vi "Main.vi"(8 "error in":errorcluster, 11 "MainUI in":refnum<class "MainUI.lvclass">) -> (0 "error out":errorcluster, 3 "MainUI out":refnum<class "MainUI.lvclass">)   [LabVIEW 2019, in "MainUI.lvclass"]
doc: "The <b>Queued Message Handler</b> of the Worker that owns this VI."
uses:
  MainUI.lvclass
  MainUI.lvclass/MainUI.ctl
  Initialization Data.ctl
  Response Cases.ctl
  rql_CallMAGetMeasureData.ctl
  rql_CallMBGetMeterValue.ctl
  rql_CallMCGetDIOStatus.ctl
  ModuleA/ModuleA.lvclass
  ModuleB/ModuleB.lvclass
  ModuleC/ModuleC.lvclass
  rql_UpdatePanel.ctl
  rql_SchduleABC.ctl
  rql_SchduleCAB.ctl
  rql_SchduleBCA.ctl
panel:
  in  "B>C>A":bool
  in  "C>A>B":bool
  in  "A>B>C":bool
  in  "ReadDIO":bool
  in  "ReadMeter":bool
  in  "ReadWaveform":bool
  out "DIOStatus":bool[](array[boolean])
  out "Meter":dbl(knob) scale=20.0..30.0
  out "Waveform Graph":waveform(dbl)(graph)
  # "讓各module 自我讀取最新數值 \n在MainUI 呼叫要求時回報最後的數據"
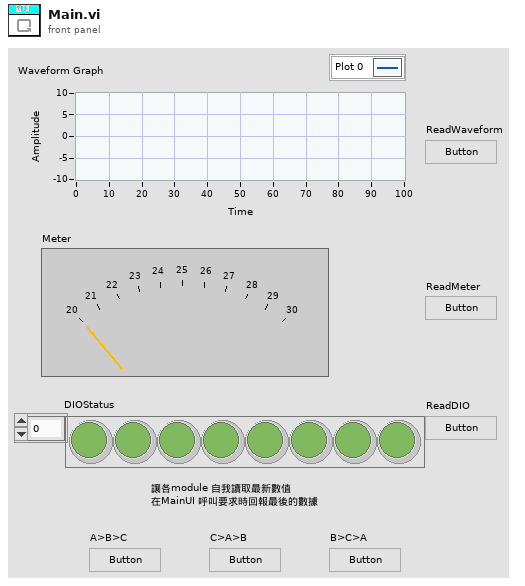
[diagram p1: front panel]
types:
  T1 = typedef "MainUI.lvclass/Initialization Data.ctl" = cluster{"Response Cases":T2}
  T2 = typedef "MainUI.lvclass/Response Cases.ctl" = cluster{"Placeholder - Can be deleted":string}
  T3 = typedef "MainUI.lvclass/rql_CallMAGetMeasureData.ctl" = cluster{"String":string}
  T4 = typedef "MainUI.lvclass/rql_CallMBGetMeterValue.ctl" = cluster{"String":string}
  T5 = typedef "MainUI.lvclass/rql_CallMCGetDIOStatus.ctl" = cluster{"String":string}
  T6 = typedef "MainUI.lvclass/rql_UpdatePanel.ctl" = cluster{"String":string}
  T7 = typedef "MainUI.lvclass/rql_SchduleABC.ctl" = cluster{"String":string}
  T8 = typedef "MainUI.lvclass/rql_SchduleCAB.ctl" = cluster{"String":string}
  T9 = typedef "MainUI.lvclass/rql_SchduleBCA.ctl" = cluster{"String":string}
  T10 = typedef "ModuleA.lvclass/rwr_RequestMeasureData Reply.ctl" = cluster{"String":string, "Waveform":waveform(dbl)}
  T11 = typedef "ModuleB.lvclass/rwr_RequestMeterValue Reply.ctl" = cluster{"String":string, "MeterValue":dbl}
  T12 = typedef "ModuleC.lvclass/rwr_RequestDIOStatus Reply.ctl" = cluster{"String":string, "DIOStatus":bool[]}
  T13 = typedef "ModuleA.lvclass/rsp_FeedbackMA_Data.ctl" = cluster{"String":string, "Waveform":waveform(dbl)}
  T14 = typedef "ModuleB.lvclass/rsp_ReturnMeterValue.ctl" = cluster{"String":string, "MeterValue":dbl}
  T15 = typedef "ModuleC.lvclass/rsp_ReturnDIOStatus.ctl" = cluster{"String":string, "DIOStatus":bool[]}
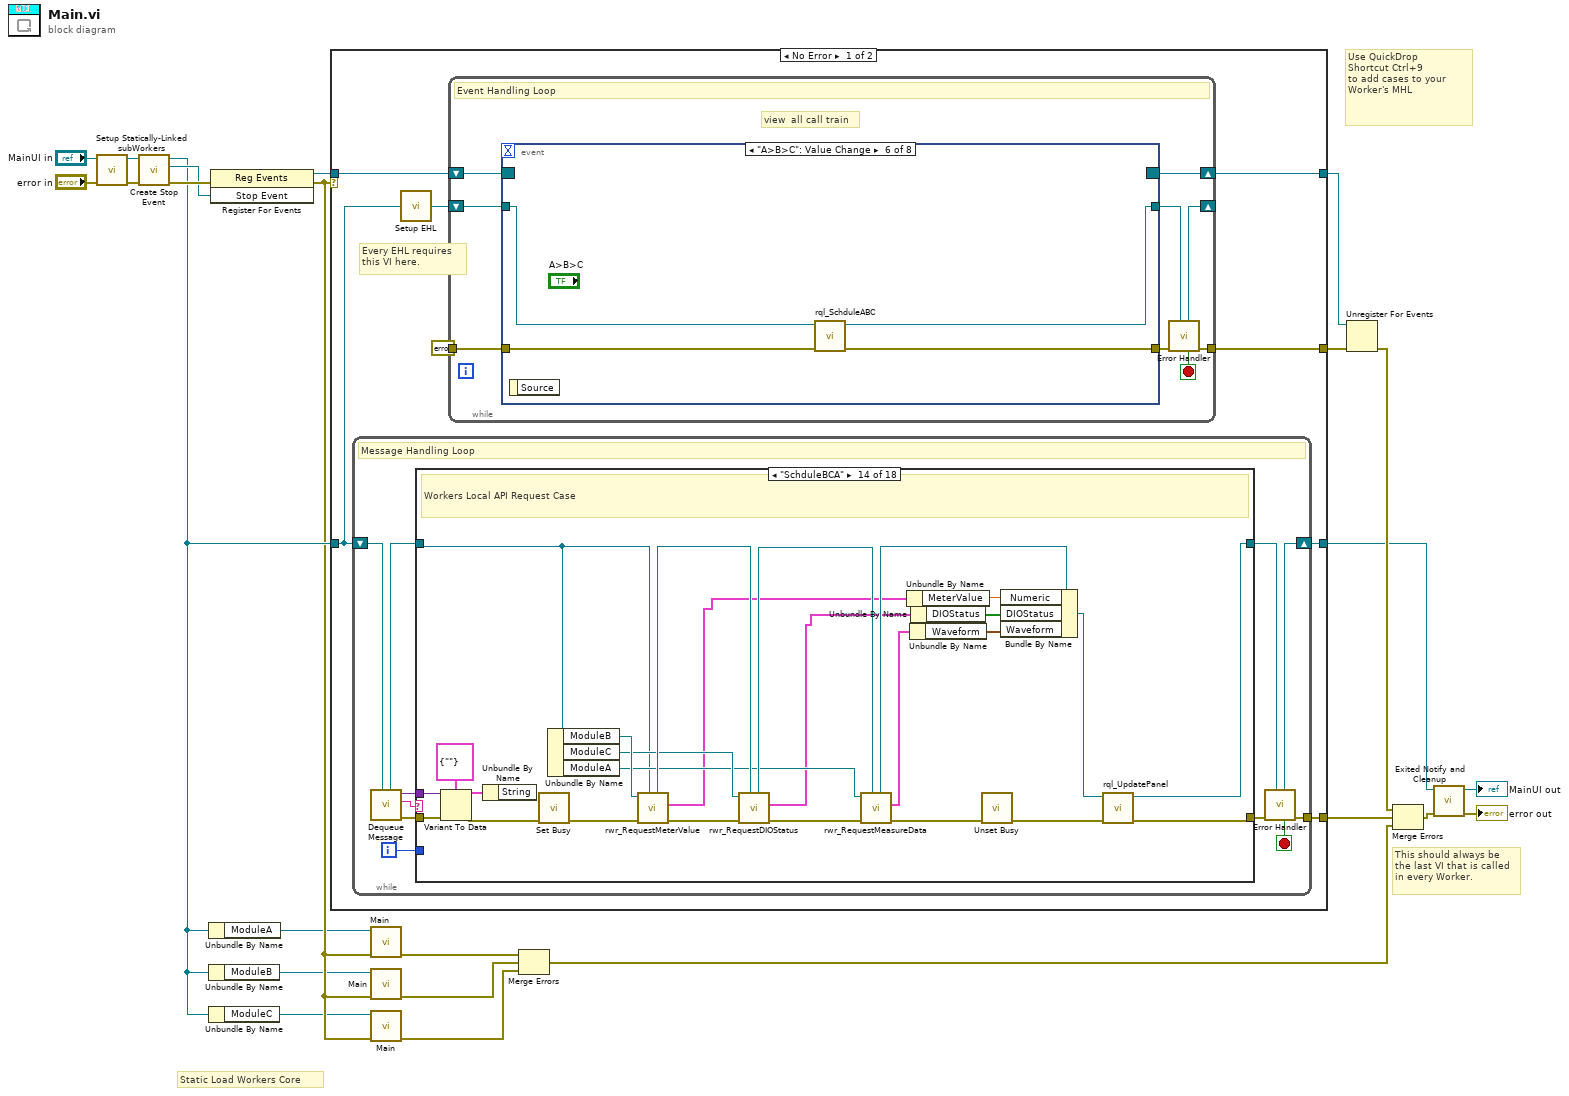
[diagram p0: block diagram]
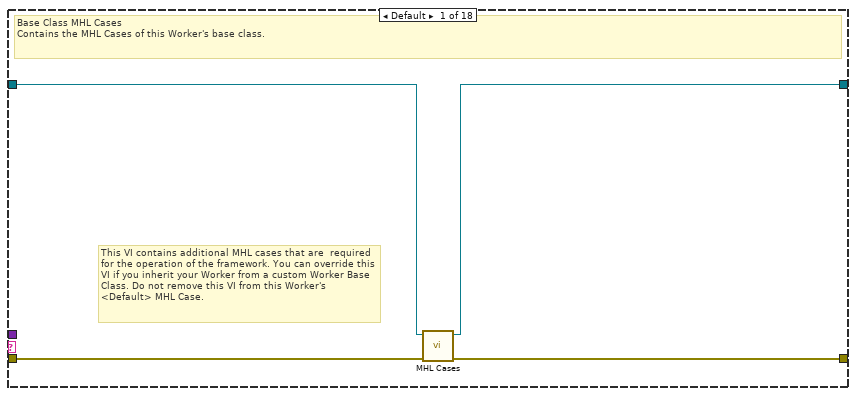
[diagram p2: hidden frame]
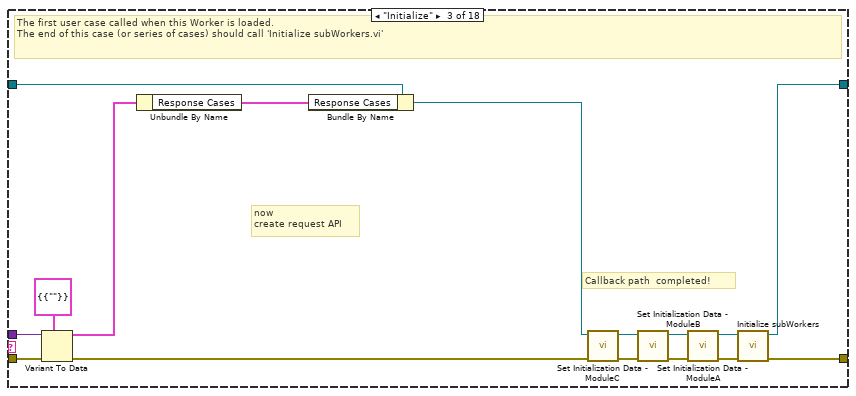
[diagram p4: hidden frame]
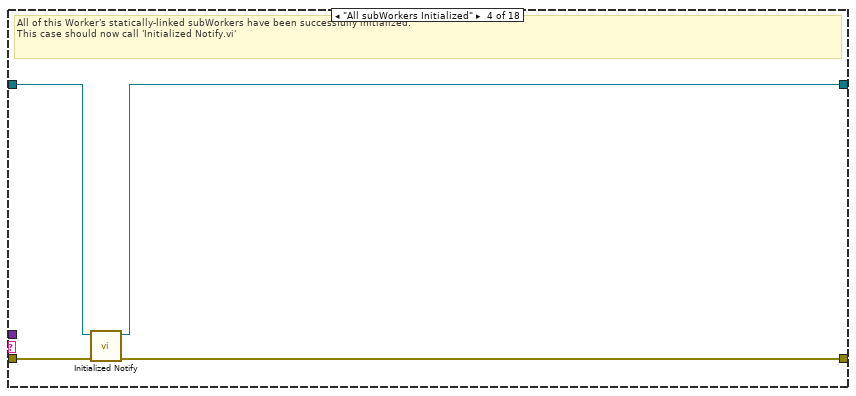
[diagram p5: hidden frame]
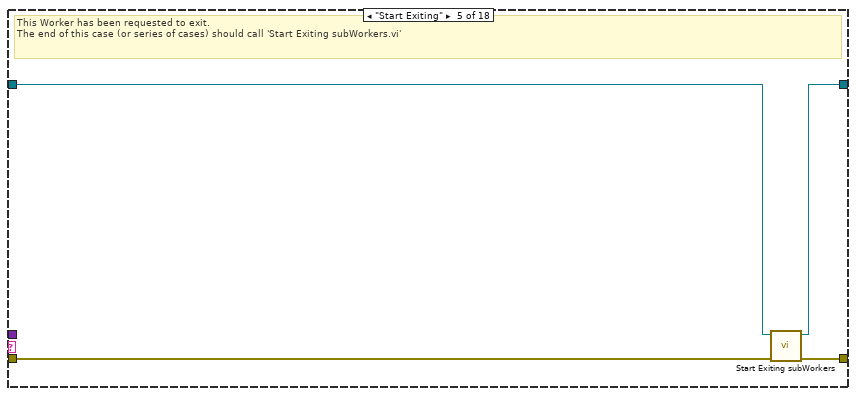
[diagram p6: hidden frame]
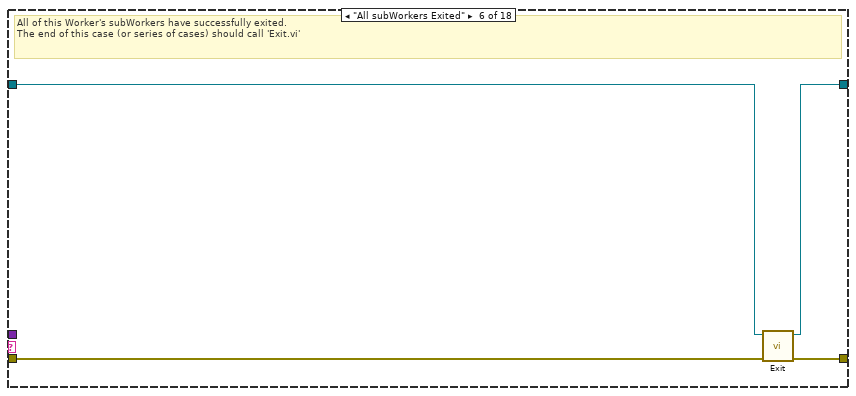
[diagram p7: hidden frame]
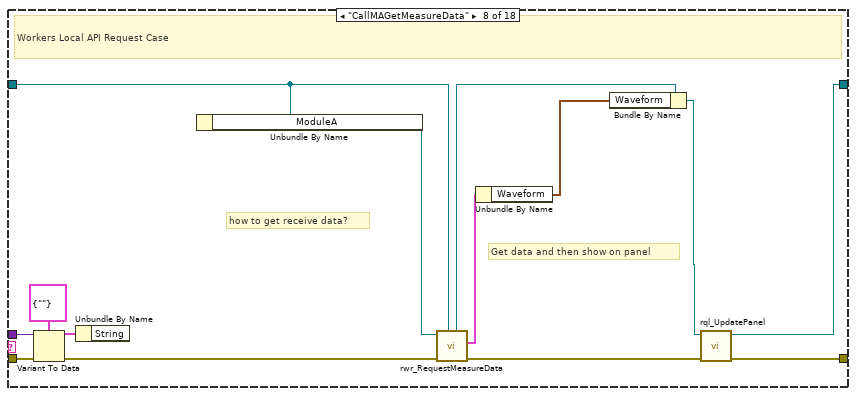
[diagram p9: hidden frame]
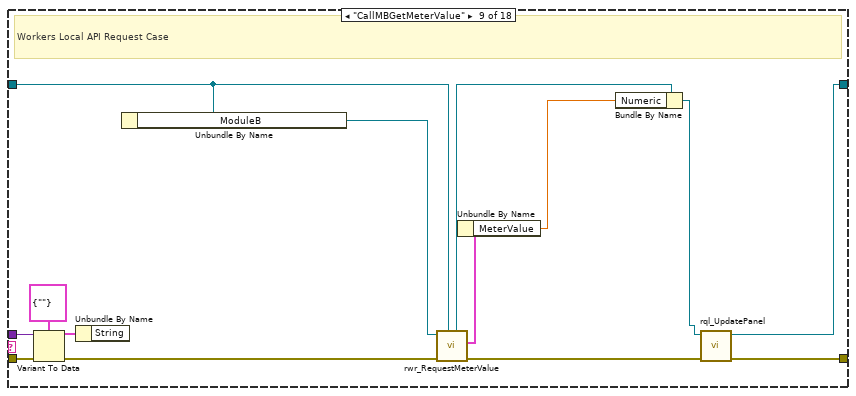
[diagram p10: hidden frame]
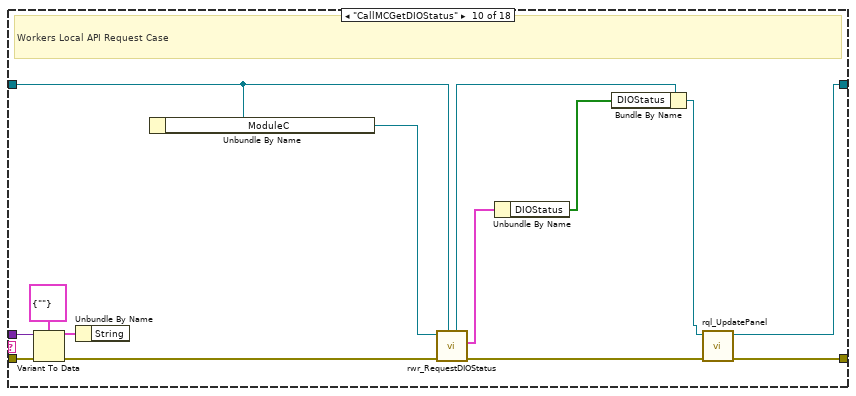
[diagram p11: hidden frame]
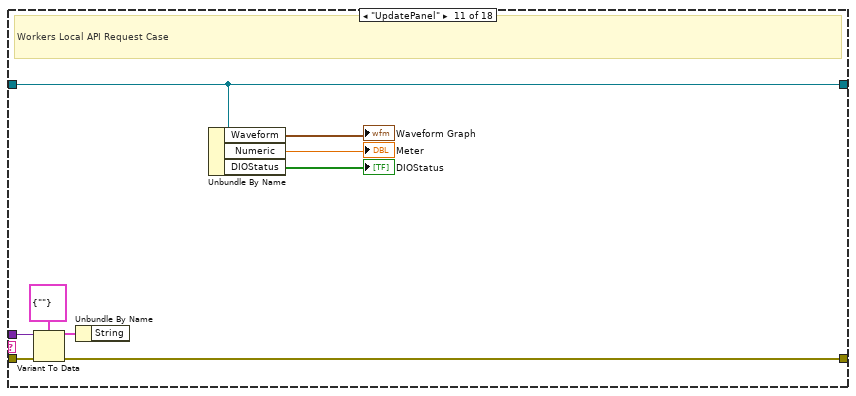
[diagram p12: hidden frame]
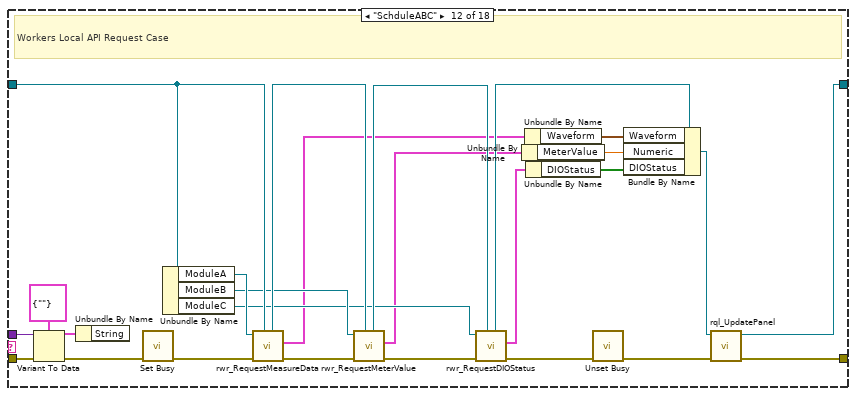
[diagram p13: hidden frame]
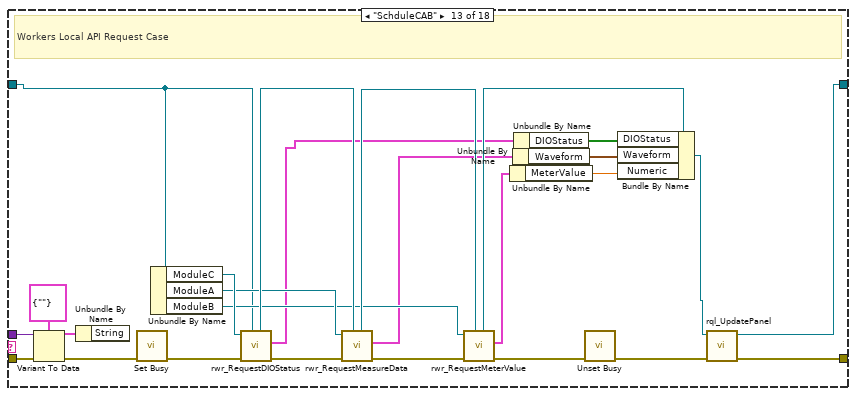
[diagram p14: hidden frame]
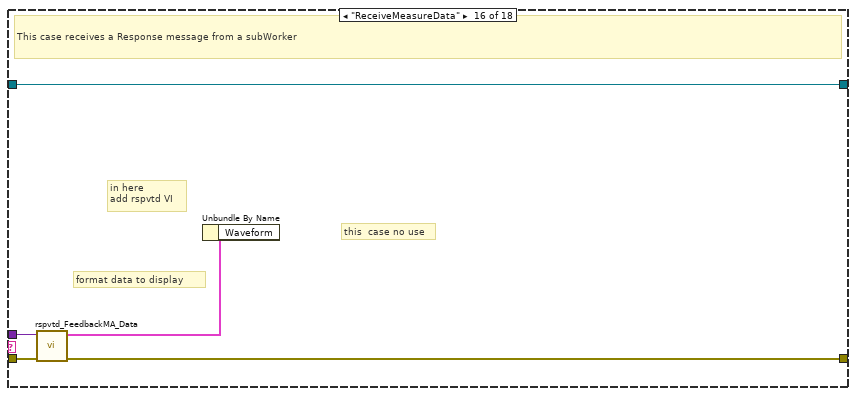
[diagram p16: hidden frame]
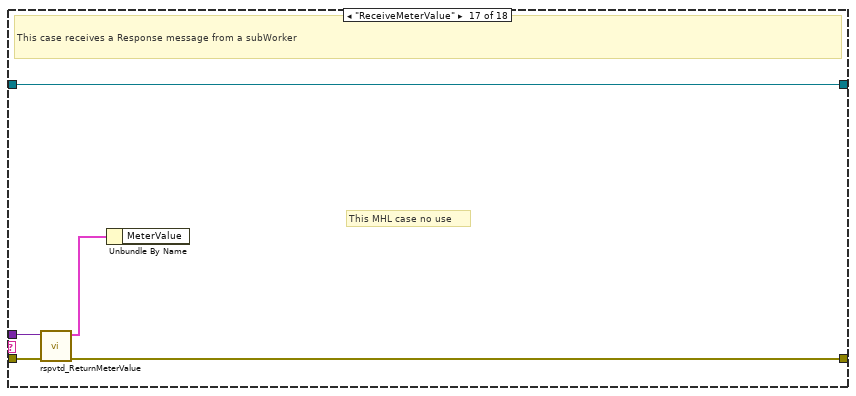
[diagram p17: hidden frame]
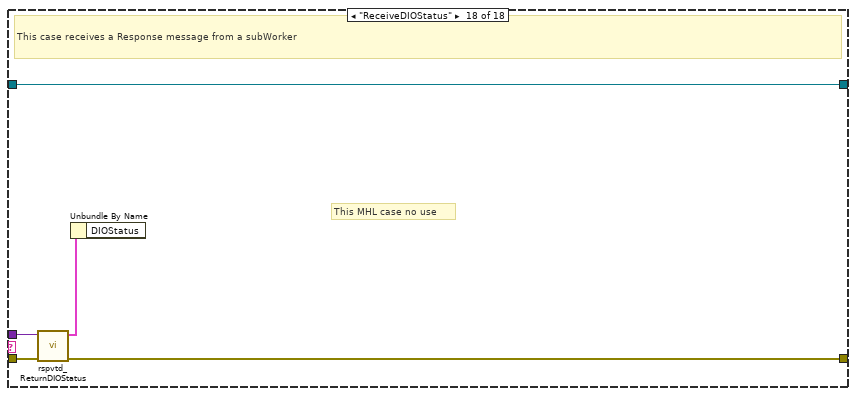
[diagram p18: hidden frame]
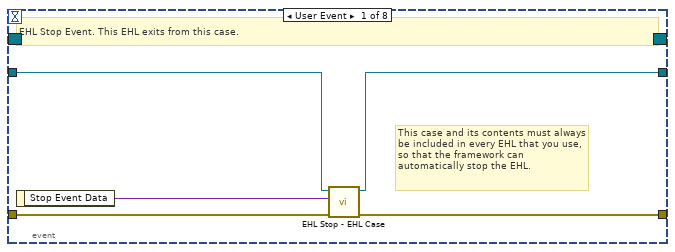
[diagram p19: hidden frame]
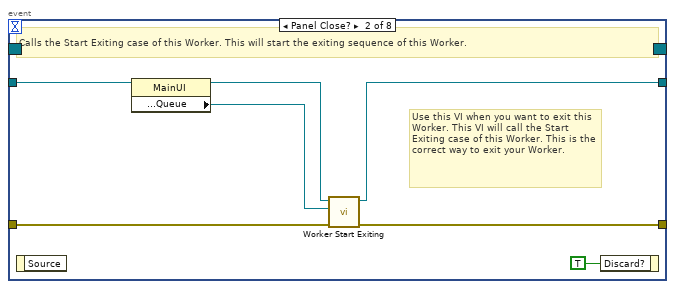
[diagram p20: hidden frame]
diagram:
  # "Static Load Workers Core"
  # "Use QuickDrop\nShortcut Ctrl+9\nto add cases to your\nWorker's MHL"
  # "This should always be the last VI that is called in every Worker."
  n1 = call "Setup Statically-Linked subWorkers.vi"("error in"="error in", "MainUI in"="MainUI in") -> ("error out"=w10:errorcluster, "MainUI out"=w8:refnum<class "MainUI.lvclass">)  [unwired: 8 in]
  n2 = call-dynamic "Create Stop Event.vi"("error in"=w10, "Worker"=w8) -> ("error out"=w19:errorcluster, "Stop Event"=w16:refnum<user-event>, "Worker out"=w13:refnum<class "MainUI.lvclass">)  [unwired: 7 in]
  n3 = Unbundle By Name(w13) -> ("ModuleA"=w5:refnum<class "ModuleA.lvclass">)
  n4 = Unbundle By Name(w13) -> ("ModuleB"=w3:refnum<class "ModuleB.lvclass">)
  n5 = Unbundle By Name(w13) -> ("ModuleC"=w1:refnum<class "ModuleC.lvclass">)
  n6 = register-events(error in=w19, w16) -> (reference out=w18:refnum<event-registration>, error out=w11:errorcluster)  [unwired: 1 in]
  n7 = case shown="No Error" w11 {
    tunnel: w13 -> [w27 w272]
    tunnel: [w25 w273] -> w17
    tunnel: w18 -> [w32 w274]
    tunnel: [w29 w275] -> w23
    tunnel: [w31 w274] -> w22
    tunnel: [w26 w271] -> w20
    selector: w11 -> [_ w275]
    frame No Error {
      # "Every EHL requires\nthis VI here."
      n8 = while {
        shift-right: [w41] -> w26
        shift-left: w27 -> [w43]
        tunnel: [w42] -> w25
        i -> [w34]
        stop <- w35 stop-if-true
        # "Message Handling Loop"
        n9 = call-dynamic "Dequeue Message.vi"("Worker"=w43) -> ("error out"=w40:errorcluster, "Case out"=w36:string, "Data out"=w33:variant, "Worker out"=w38:refnum<class "MainUI.lvclass">)  [unwired: 6 in, 1 out]
        n10 = case "Worker MHL Case Structure (DO NOT CHANGE LABEL NAME)" shown="\"SchduleBCA\"" w36 {
          tunnel: w40 -> [w47 w48 w63 w67 w70 w77 w79 w93 w107 w121 w130 w156 w182 w208 w210 w215 w220 w225]
          tunnel: [w46 w48 w65 w66 w73 w76 w79 w82 w96 w110 w129 w135 w161 w187 w210 w213 w218 w223] -> w39
          tunnel: w38 -> [w45 w49 w62 w69 w71 w75 w78 w86 w100 w114 w125 w150 w170 w196 w209 w214 w219 w224]
          tunnel: [w44 w49 w64 w68 w72 w74 w78 w80 w94 w108 w125 w133 w159 w185 w209 w214 w219 w224] -> w37
          tunnel: w34 -> [_ _ _ _ _ _ _ _ _ _ _ _ _ _ _ _ _ _]
          tunnel: w33 -> [_ _ w60 _ _ _ _ w90 w104 w118 w127 w153 w180 w206 _ w212 w217 w222]
          frame Default {
            # "This VI contains additional MHL cases that are  required for the operation of the framework. You can override this VI if you inherit your Worker from a custom Worker Base Class. Do not remove this VI from this Worker's <Default> MHL Case."
            # "Base Class MHL Cases\nContains the MHL Cases of this Worker's base class."
            n11 = call-dynamic "MHL Cases.vi"("error in"=w47, "Worker in"=w45) -> ("error out"=w46:errorcluster, "Worker out"=w44:refnum<class "MainUI.lvclass">)  [unwired: 8 in]
          }
          frame "------------ FRAMEWORK CASES -----------" {
            # "Start of Workers Framework Cases"
          }
          frame "Initialize" {
            # "now \ncreate request API"
            # "Callback path  completed!"
            # "The first user case called when this Worker is loaded.\nThe end of this case (or series of cases) should call 'Initialize subWorkers.vi'"
            n12 = Variant To Data(error in=w63, type=T1 {"Response Cases"={"Placeholder - Can be deleted"=""}} ("Initialization Data"), Variant=w60) -> (data=w59:T1, error out=w61:errorcluster)
            n13 = Unbundle By Name(w59) -> ("Response Cases"=w58:T2)
            n14 = Bundle By Name(cluster=w62, "Response Cases"=w58) -> (w51:refnum<class "MainUI.lvclass">)
            n15 = call "Set Initialization Data - ModuleC.vi"("error in"=w61, "MainUI in"=w51) -> ("error out"=w52:errorcluster, "MainUI out"=w50:refnum<class "MainUI.lvclass">)  [unwired: 8 in]
            n16 = call "Set Initialization Data - ModuleB.vi"("error in"=w52, "MainUI in"=w50) -> ("error out"=w54:errorcluster, "MainUI out"=w53:refnum<class "MainUI.lvclass">)  [unwired: 8 in]
            n17 = call "Set Initialization Data - ModuleA.vi"("error in"=w54, "MainUI in"=w53) -> ("error out"=w56:errorcluster, "MainUI out"=w55:refnum<class "MainUI.lvclass">)  [unwired: 8 in]
            n18 = call-dynamic "Initialize subWorkers.vi"("error in"=w56, "Worker"=w55) -> ("error out"=w65:errorcluster, "dup Worker out"=w64:refnum<class "MainUI.lvclass">)  [unwired: 8 in]
          }
          frame "All subWorkers Initialized" {
            # "All of this Worker's statically-linked subWorkers have been successfully initialized.\nThis case should now call 'Initialized Notify.vi'"
            n19 = call-dynamic "Initialized Notify.vi"("error in"=w67, "Worker"=w69) -> ("error out"=w66:errorcluster, "dup Worker out"=w68:refnum<class "MainUI.lvclass">)  [unwired: 8 in]
          }
          frame "Start Exiting" {
            # "This Worker has been requested to exit. \nThe end of this case (or series of cases) should call 'Start Exiting subWorkers.vi'"
            n20 = call-dynamic "Start Exiting subWorkers.vi"("error_in"=w70, "Worker"=w71) -> ("error out"=w73:errorcluster, "dup Worker out"=w72:refnum<class "MainUI.lvclass">)  [unwired: 8 in]
          }
          frame "All subWorkers Exited" {
            # "All of this Worker's subWorkers have successfully exited. \nThe end of this case (or series of cases) should call 'Exit.vi'"
            n21 = call-dynamic "Exit.vi"("error_in"=w77, "Worker"=w75) -> ("error out"=w76:errorcluster, "dup Worker out"=w74:refnum<class "MainUI.lvclass">)  [unwired: 8 in]
          }
          frame "------------- LOCAL API CASES -------------" {
            # "Start of Workers Local API Cases"
          }
          frame "CallMAGetMeasureData" {
            # "Get data and then show on panel"
            # "how to get receive data?"
            # "Workers Local API Request Case"
            n22 = Variant To Data(error in=w93, type=T3 {"String"=""} ("Data"), Variant=w90) -> (data=w89:T3, error out=w92:errorcluster)
            n23 = Unbundle By Name(w89) -> ()  [unwired: 1 out]
            n24 = Unbundle By Name(w86) -> ("ModuleA"=w85:refnum<class "ModuleA.lvclass">)
            n25 = call "rwr_RequestMeasureData.vi"("Caller in"=w86, "error in"=w92, "ModuleA in"=w85) -> ("error out"=w88:errorcluster, "Reply Data out"=w84:T10, "dup Caller out"=w87:refnum<class "MainUI.lvclass">)  [unwired: 5 in, 1 out]
            n26 = Unbundle By Name(w84) -> ("Waveform"=w83:waveform(dbl))
            n27 = Bundle By Name(cluster=w87, "Waveform"=w83) -> (w81:refnum<class "MainUI.lvclass">)
            n28 = call "rql_UpdatePanel.vi"("error in"=w88, "MainUI in"=w81) -> ("error out"=w82:errorcluster, "dup MainUI out"=w80:refnum<class "MainUI.lvclass">)  [unwired: 8 in]
          }
          frame "CallMBGetMeterValue" {
            # "Workers Local API Request Case"
            n29 = Variant To Data(error in=w107, type=T4 {"String"=""} ("Data"), Variant=w104) -> (data=w103:T4, error out=w106:errorcluster)
            n30 = Unbundle By Name(w103) -> ()  [unwired: 1 out]
            n31 = Unbundle By Name(w100) -> ("ModuleB"=w99:refnum<class "ModuleB.lvclass">)
            n32 = call "rwr_RequestMeterValue.vi"("Caller in"=w100, "error in"=w106, "ModuleB in"=w99) -> ("error out"=w102:errorcluster, "Reply Data out"=w98:T11, "dup Caller out"=w101:refnum<class "MainUI.lvclass">)  [unwired: 5 in, 1 out]
            n33 = Unbundle By Name(w98) -> ("MeterValue"=w97:dbl)
            n34 = Bundle By Name(cluster=w101, "Numeric"=w97) -> (w95:refnum<class "MainUI.lvclass">)
            n35 = call "rql_UpdatePanel.vi"("error in"=w102, "MainUI in"=w95) -> ("error out"=w96:errorcluster, "dup MainUI out"=w94:refnum<class "MainUI.lvclass">)  [unwired: 8 in]
          }
          frame "CallMCGetDIOStatus" {
            # "Workers Local API Request Case"
            n36 = Variant To Data(error in=w121, type=T5 {"String"=""} ("Data"), Variant=w118) -> (data=w117:T5, error out=w120:errorcluster)
            n37 = Unbundle By Name(w117) -> ()  [unwired: 1 out]
            n38 = Unbundle By Name(w114) -> ("ModuleC"=w113:refnum<class "ModuleC.lvclass">)
            n39 = call "rwr_RequestDIOStatus.vi"("Caller in"=w114, "error in"=w120, "ModuleC in"=w113) -> ("error out"=w116:errorcluster, "Reply Data out"=w112:T12, "dup Caller out"=w115:refnum<class "MainUI.lvclass">)  [unwired: 5 in, 1 out]
            n40 = Unbundle By Name(w112) -> ("DIOStatus"=w111:bool[])
            n41 = Bundle By Name(cluster=w115, "DIOStatus"=w111) -> (w109:refnum<class "MainUI.lvclass">)
            n42 = call "rql_UpdatePanel.vi"("error in"=w116, "MainUI in"=w109) -> ("error out"=w110:errorcluster, "dup MainUI out"=w108:refnum<class "MainUI.lvclass">)  [unwired: 8 in]
          }
          frame "UpdatePanel" {
            # "Workers Local API Request Case"
            n43 = Variant To Data(error in=w130, type=T6 {"String"=""} ("Data"), Variant=w127) -> (data=w126:T6, error out=w129:errorcluster)
            n44 = Unbundle By Name(w126) -> ()  [unwired: 1 out]
            n45 = Unbundle By Name(w125) -> ("Waveform"=→"Waveform Graph":waveform(dbl), "Numeric"=→"Meter":dbl, "DIOStatus"=→"DIOStatus":bool[])
          }
          frame "SchduleABC" {
            # "Workers Local API Request Case"
            n46 = Variant To Data(error in=w156, type=T7 {"String"=""} ("Data"), Variant=w153) -> (data=w152:T7, error out=w155:errorcluster)
            n47 = Unbundle By Name(w152) -> ()  [unwired: 1 out]
            n48 = call <vilib>:"Set Busy.vi"("error in (no error)"=w155) -> ("error out"=w132:errorcluster)  [unwired: 9 in, 1 out]
            n49 = Unbundle By Name(w150) -> ("ModuleA"=w149:refnum<class "ModuleA.lvclass">, "ModuleB"=w146:refnum<class "ModuleB.lvclass">, "ModuleC"=w142:refnum<class "ModuleC.lvclass">)
            n50 = call "rwr_RequestMeasureData.vi"("Caller in"=w150, "error in"=w132, "ModuleA in"=w149) -> ("error out"=w151:errorcluster, "Reply Data out"=w141:T10, "dup Caller out"=w147:refnum<class "MainUI.lvclass">)  [unwired: 5 in, 1 out]
            n51 = call "rwr_RequestMeterValue.vi"("Caller in"=w147, "error in"=w151, "ModuleB in"=w146) -> ("error out"=w148:errorcluster, "Reply Data out"=w140:T11, "dup Caller out"=w144:refnum<class "MainUI.lvclass">)  [unwired: 5 in, 1 out]
            n52 = call "rwr_RequestDIOStatus.vi"("Caller in"=w144, "error in"=w148, "ModuleC in"=w142) -> ("error out"=w145:errorcluster, "Reply Data out"=w139:T12, "dup Caller out"=w143:refnum<class "MainUI.lvclass">)  [unwired: 5 in, 1 out]
            n53 = Unbundle By Name(w140) -> ("MeterValue"=w137:dbl)
            n54 = Unbundle By Name(w141) -> ("Waveform"=w138:waveform(dbl))
            n55 = Unbundle By Name(w139) -> ("DIOStatus"=w136:bool[])
            n56 = call <vilib>:"Unset Busy.vi"("error in (no error)"=w145) -> ("error out"=w131:errorcluster)  [unwired: 10 in]
            n57 = Bundle By Name(cluster=w143, "Waveform"=w138, "Numeric"=w137, "DIOStatus"=w136) -> (w134:refnum<class "MainUI.lvclass">)
            n58 = call "rql_UpdatePanel.vi"("error in"=w131, "MainUI in"=w134) -> ("error out"=w135:errorcluster, "dup MainUI out"=w133:refnum<class "MainUI.lvclass">)  [unwired: 8 in]
          }
          frame "SchduleCAB" {
            # "Workers Local API Request Case"
            n59 = Variant To Data(error in=w182, type=T8 {"String"=""} ("Data"), Variant=w180) -> (data=w179:T8, error out=w169:errorcluster)
            n60 = Unbundle By Name(w179) -> ()  [unwired: 1 out]
            n61 = call <vilib>:"Set Busy.vi"("error in (no error)"=w169) -> ("error out"=w158:errorcluster)  [unwired: 9 in, 1 out]
            n62 = Unbundle By Name(w170) -> ("ModuleC"=w177:refnum<class "ModuleC.lvclass">, "ModuleA"=w174:refnum<class "ModuleA.lvclass">, "ModuleB"=w171:refnum<class "ModuleB.lvclass">)
            n63 = call "rwr_RequestDIOStatus.vi"("Caller in"=w170, "error in"=w158, "ModuleC in"=w177) -> ("error out"=w178:errorcluster, "Reply Data out"=w167:T12, "dup Caller out"=w175:refnum<class "MainUI.lvclass">)  [unwired: 5 in, 1 out]
            n64 = call "rwr_RequestMeasureData.vi"("Caller in"=w175, "error in"=w178, "ModuleA in"=w174) -> ("error out"=w176:errorcluster, "Reply Data out"=w166:T10, "dup Caller out"=w173:refnum<class "MainUI.lvclass">)  [unwired: 5 in, 1 out]
            n65 = call "rwr_RequestMeterValue.vi"("Caller in"=w173, "error in"=w176, "ModuleB in"=w171) -> ("error out"=w168:errorcluster, "Reply Data out"=w165:T11, "dup Caller out"=w172:refnum<class "MainUI.lvclass">)  [unwired: 5 in, 1 out]
            n66 = Unbundle By Name(w165) -> ("MeterValue"=w164:dbl)
            n67 = Unbundle By Name(w166) -> ("Waveform"=w163:waveform(dbl))
            n68 = Unbundle By Name(w167) -> ("DIOStatus"=w162:bool[])
            n69 = call <vilib>:"Unset Busy.vi"("error in (no error)"=w168) -> ("error out"=w157:errorcluster)  [unwired: 10 in]
            n70 = Bundle By Name(cluster=w172, "DIOStatus"=w162, "Waveform"=w163, "Numeric"=w164) -> (w160:refnum<class "MainUI.lvclass">)
            n71 = call "rql_UpdatePanel.vi"("error in"=w157, "MainUI in"=w160) -> ("error out"=w161:errorcluster, "dup MainUI out"=w159:refnum<class "MainUI.lvclass">)  [unwired: 8 in]
          }
          frame "SchduleBCA" {
            # "Workers Local API Request Case"
            n72 = Variant To Data(error in=w208, type=T9 {"String"=""} ("Data"), Variant=w206) -> (data=w205:T9, error out=w195:errorcluster)
            n73 = Unbundle By Name(w205) -> ()  [unwired: 1 out]
            n74 = call <vilib>:"Set Busy.vi"("error in (no error)"=w195) -> ("error out"=w184:errorcluster)  [unwired: 9 in, 1 out]
            n75 = Unbundle By Name(w196) -> ("ModuleB"=w203:refnum<class "ModuleB.lvclass">, "ModuleC"=w200:refnum<class "ModuleC.lvclass">, "ModuleA"=w197:refnum<class "ModuleA.lvclass">)
            n76 = call "rwr_RequestMeterValue.vi"("Caller in"=w196, "error in"=w184, "ModuleB in"=w203) -> ("error out"=w204:errorcluster, "Reply Data out"=w193:T11, "dup Caller out"=w201:refnum<class "MainUI.lvclass">)  [unwired: 5 in, 1 out]
            n77 = call "rwr_RequestDIOStatus.vi"("Caller in"=w201, "error in"=w204, "ModuleC in"=w200) -> ("error out"=w202:errorcluster, "Reply Data out"=w192:T12, "dup Caller out"=w199:refnum<class "MainUI.lvclass">)  [unwired: 5 in, 1 out]
            n78 = call "rwr_RequestMeasureData.vi"("Caller in"=w199, "error in"=w202, "ModuleA in"=w197) -> ("error out"=w194:errorcluster, "Reply Data out"=w191:T10, "dup Caller out"=w198:refnum<class "MainUI.lvclass">)  [unwired: 5 in, 1 out]
            n79 = Unbundle By Name(w193) -> ("MeterValue"=w190:dbl)
            n80 = Unbundle By Name(w191) -> ("Waveform"=w188:waveform(dbl))
            n81 = Unbundle By Name(w192) -> ("DIOStatus"=w189:bool[])
            n82 = call <vilib>:"Unset Busy.vi"("error in (no error)"=w194) -> ("error out"=w183:errorcluster)  [unwired: 10 in]
            n83 = Bundle By Name(cluster=w198, "Numeric"=w190, "DIOStatus"=w189, "Waveform"=w188) -> (w186:refnum<class "MainUI.lvclass">)
            n84 = call "rql_UpdatePanel.vi"("error in"=w183, "MainUI in"=w186) -> ("error out"=w187:errorcluster, "dup MainUI out"=w185:refnum<class "MainUI.lvclass">)  [unwired: 8 in]
          }
          frame "------------- RESPONSE CASES --------------" {
            # "Start of Workers Response Cases"
          }
          frame "ReceiveMeasureData" {
            # "this  case no use"
            # "format data to display"
            # "in here \nadd rspvtd VI"
            # "This case receives a Response message from a subWorker"
            n85 = call "rspvtd_FeedbackMA_Data.vi"("error in"=w215, "Data in"=w212) -> ("error out"=w213:errorcluster, "Data out"=w211:T13)  [unwired: 8 in]
            n86 = Unbundle By Name(w211) -> ()  [unwired: 1 out]
          }
          frame "ReceiveMeterValue" {
            # "This MHL case no use"
            # "This case receives a Response message from a subWorker"
            n87 = call "rspvtd_ReturnMeterValue.vi"("error in"=w220, "Data in"=w217) -> ("error out"=w218:errorcluster, "Data out"=w216:T14)  [unwired: 8 in]
            n88 = Unbundle By Name(w216) -> ()  [unwired: 1 out]
          }
          frame "ReceiveDIOStatus" {
            # "This MHL case no use"
            # "This case receives a Response message from a subWorker"
            n89 = call "rspvtd_ReturnDIOStatus.vi"("error in"=w225, "Data in"=w222) -> ("error out"=w223:errorcluster, "Data out"=w221:T15)  [unwired: 8 in]
            n90 = Unbundle By Name(w221) -> ()  [unwired: 1 out]
          }
        }
        n91 = call-dynamic "Error Handler.vi"("Worker"=w37, "error_in"=w39) -> ("error out"=w42:errorcluster, "Stop Loop"=w35:bool, "Worker out"=w41:refnum<class "MainUI.lvclass">)  [unwired: 7 in]
      }
      n92 = call-dynamic "Setup EHL.vi"("Worker"=w27) -> ("Worker out"=w28:refnum<class "MainUI.lvclass">)  [unwired: 14 in]
      n93 = while "Event Handling Loop" {
        shift-right: [w234] -> w31
        shift-left: w32 -> [w233]
        tunnel: [w229] -> w29
        tunnel: errorcluster {"status"=FALSE, "code"=0, "source"=""} ("error constant") -> [w231]
        shift-right: [w227] -> _
        shift-left: w28 -> [w232]
        stop <- w226 stop-if-true
        # "view  all call train"
        # "Event Handling Loop"
        n94 = event shown="[5] \"A>B>C\": Value Change" {
          selector: w233 -> [_ _ _ _ _ _ _ _]
          dyn-events: [_ _ _ _ _ _ _ _] -> w234
          timeout: _ -> [_ _ _ _ _ _ _ _]
          tunnel: [w238 w245 w249 w253 w257 w261 w265 w269] -> w230
          tunnel: w231 -> [w239 w244 w250 w254 w258 w262 w266 w270]
          tunnel: w232 -> [w237 w243 w248 w252 w256 w260 w264 w268]
          tunnel: [w236 w242 w247 w251 w255 w259 w263 w267] -> w228
          event User Event {
            # "This case and its contents must always be included in every EHL that you use, so that the framework can automatically stop the EHL."
            # "EHL Stop Event. This EHL exits from this case."
            n95 = event-data() -> ("Stop Event Data"=w235:variant)  [unwired: 1 in]
            n96 = call-dynamic "EHL Stop - EHL Case.vi"("error in"=w239, "Stop Event Data"=w235, "Worker"=w237) -> ("error out"=w238:errorcluster, "Worker out"=w236:refnum<class "MainUI.lvclass">)  [unwired: 7 in]
          }
          event Panel Close? {
            # "Use this VI when you want to exit this Worker. This VI will call the Start Exiting case of this Worker. This is the correct way to exit your Worker."
            # "Calls the Start Exiting case of this Worker. This will start the exiting sequence of this Worker."
            n97 = event-data() -> ()  [unwired: 1 in, 1 out]
            n98 = property class="MainUI"(reference=w243) -> (reference out=w241:refnum<class "MainUI.lvclass">, "Accessors:Read:Public API:Queue"=w240:refnum<class "Message Queue.lvclass">)  [unwired: 1 in, 1 out]
            n99 = call-dynamic "Worker Start Exiting.vi"("error_in"=w244, "Message Queue"=w240, "Worker"=w241) -> ("error out"=w245:errorcluster, "dup Worker out"=w242:refnum<class "MainUI.lvclass">)  [unwired: 7 in]
            n100 = event-data ("Event Filter Node")("Discard?"=TRUE) -> ()  [unwired: 1 in, 1 out]
          }
          event "ReadWaveform": Value Change {
            n101 = event-data() -> ()  [unwired: 1 in, 1 out]
            n102 = call "rql_CallMAGetMeasureData.vi"("error in"=w250, "MainUI in"=w248) -> ("error out"=w249:errorcluster, "dup MainUI out"=w247:refnum<class "MainUI.lvclass">)  [unwired: 8 in]
          }
          event "ReadMeter": Value Change {
            n103 = event-data() -> ()  [unwired: 1 in, 1 out]
            n104 = call "rql_CallMBGetMeterValue.vi"("error in"=w254, "MainUI in"=w252) -> ("error out"=w253:errorcluster, "dup MainUI out"=w251:refnum<class "MainUI.lvclass">)  [unwired: 8 in]
          }
          event "ReadDIO": Value Change {
            n105 = event-data() -> ()  [unwired: 1 in, 1 out]
            n106 = call "rql_CallMCGetDIOStatus.vi"("error in"=w258, "MainUI in"=w256) -> ("error out"=w257:errorcluster, "dup MainUI out"=w255:refnum<class "MainUI.lvclass">)  [unwired: 8 in]
          }
          event "A>B>C": Value Change {
            n107 = event-data() -> ()  [unwired: 1 in, 1 out]
            n108 = call "rql_SchduleABC.vi"("error in"=w262, "MainUI in"=w260) -> ("error out"=w261:errorcluster, "dup MainUI out"=w259:refnum<class "MainUI.lvclass">)  [unwired: 8 in]
          }
          event "C>A>B": Value Change {
            n109 = event-data() -> ()  [unwired: 1 in, 1 out]
            n110 = call "rql_SchduleCAB.vi"("error in"=w266, "MainUI in"=w264) -> ("error out"=w265:errorcluster, "dup MainUI out"=w263:refnum<class "MainUI.lvclass">)  [unwired: 8 in]
          }
          event "B>C>A": Value Change {
            n111 = event-data() -> ()  [unwired: 1 in, 1 out]
            n112 = call "rql_SchduleBCA.vi"("error in"=w270, "MainUI in"=w268) -> ("error out"=w269:errorcluster, "dup MainUI out"=w267:refnum<class "MainUI.lvclass">)  [unwired: 8 in]
          }
        }
        n113 = call-dynamic "Error Handler.vi"("Worker"=w228, "error_in"=w230) -> ("error out"=w229:errorcluster, "Stop Loop"=w226:bool, "Worker out"=w227:refnum<class "MainUI.lvclass">)  [unwired: 7 in]
      }
    }
    frame Error {
      n114 = call-dynamic "Error Handler.vi"("Worker"=w272, "error_in"=w275) -> ("error out"=w273:errorcluster, "Worker out"=w271:refnum<class "MainUI.lvclass">)  [unwired: 7 in, 1 out]
    }
  }
  n115 = call-dynamic "Main.vi"("error in"=w11, "ModuleA in"=w5) -> ("error out"=w7:errorcluster)  [unwired: 8 in, 1 out]
  n116 = call-dynamic "Main.vi"("error in"=w11, "ModuleB in"=w3) -> ("error out"=w4:errorcluster)  [unwired: 8 in, 1 out]
  n117 = call-dynamic "Main.vi"("error in"=w11, "ModuleC in"=w1) -> ("error out"=w2:errorcluster)  [unwired: 8 in, 1 out]
  n118 = Merge Errors(w7, w4, w2) -> (w6:errorcluster)
  n119 = Unregister For Events(event registration refnum=w22, error in=w23) -> (error out=w24:errorcluster)
  n120 = Merge Errors(w24, w17, w6) -> (w21:errorcluster)
  n121 = call-dynamic "Exited Notify and Cleanup.vi"("error_in"=w21, "Worker"=w20) -> ("error out"=→"error out":errorcluster, "dup Worker out"=→"MainUI out":refnum<class "MainUI.lvclass">)  [unwired: 8 in]
